vi "Mask (SubVI).vi"(10 "pulse duration[sample]":i8, 11 "M":i8) -> (3 "Array":dbl[][](array[numeric]))   [LabVIEW 2017]
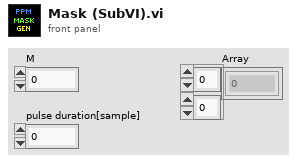
[diagram p1: front panel]
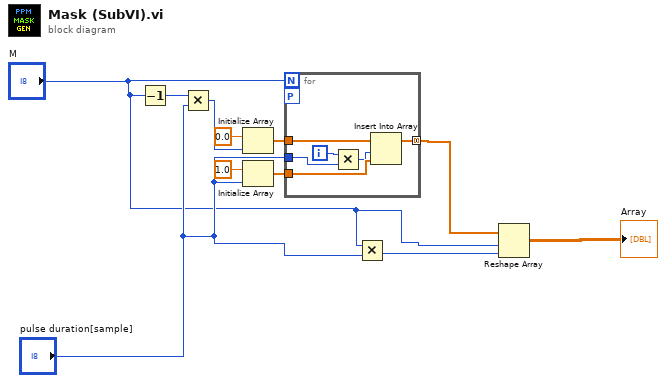
[diagram p0: block diagram]
diagram:
  n1 = Decrement(x="M") -> (x-1=w6:i8)
  n2 = Multiply(x=w6, y="pulse duration[sample]") -> (x*y=w3:i8)
  n3 = Initialize Array(0.0 ("element"), w3) -> (w4:dbl[])
  n4 = Initialize Array(1.0 ("element"), "pulse duration[sample]") -> (w5:dbl[])
  n5 = for {
    N: "M" -> [_]
    tunnel: w4 -> [w17]
    tunnel: w5 -> [w16]
    tunnel: [w15] -> w9 mode=concatenating
    tunnel: "pulse duration[sample]" -> [w14]
    workers-P: _ -> [_]
    i -> [w12]
    n6 = Multiply(x=w12, y=w14) -> (x*y=w13:i32)
    n7 = Insert Into Array(array=w17, index=w13, new element=w16) -> (w15:dbl[])
  }
  n8 = Multiply(x="M", y="pulse duration[sample]") -> (x*y=w7:i8)
  n9 = Reshape Array(w9, "M", w7) -> (→"Array":dbl[][])
